vi "CTRE_Phoenix_CANCoder_GetVelocity.vi"(8 "error in":errorcluster, 11 "CTRE_CANcoder_DeviceRef":T1) -> (0 "error out":errorcluster, 2 "Velocity":dbl format="%.2f", 3 "CTRE_CANcoder_DeviceRef":T1)   [LabVIEW 2019]
doc: "Returns the velocity of the CANcoder."
uses:
  <vilib>/Rock Robotics/WPI/ThirdParty/Phoenix-LabVIEW/CANCoder/Controls/CTRE_Phoenix_CANcoder_DeviceRef.ctl
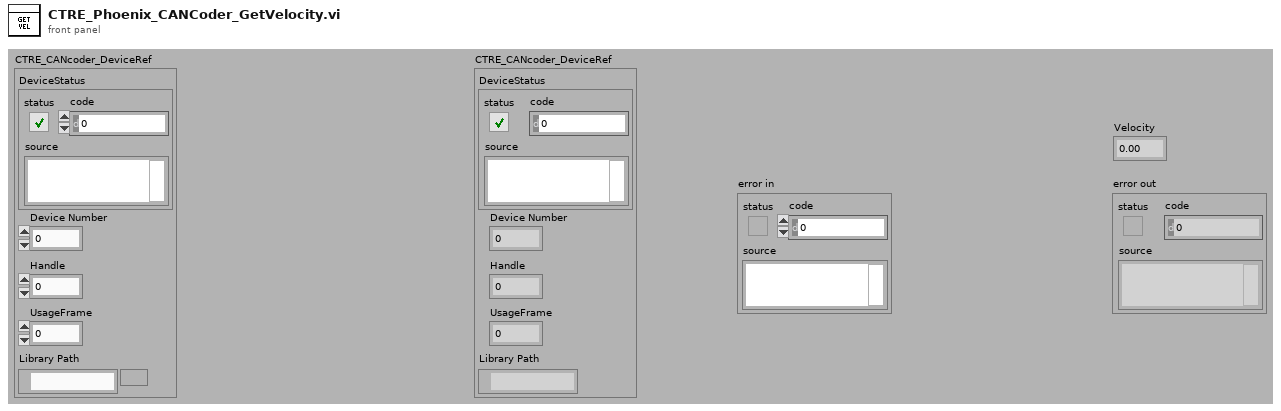
[diagram p1: front panel]
types:
  T1 = typedef "CTRE_Phoenix_CANcoder_DeviceRef.ctl" = cluster{"DeviceStatus":errorcluster, "Device Number":u8, "Handle":u64, "UsageFrame":u32, "Library Path":path}
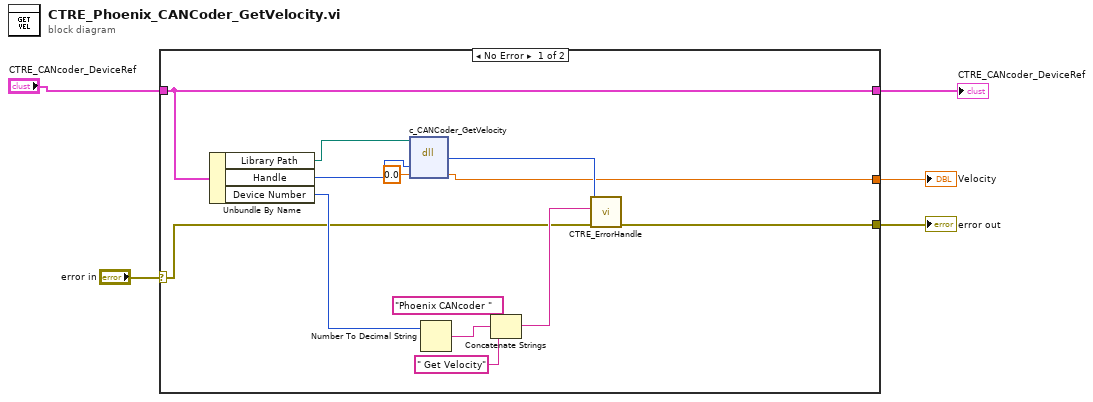
[diagram p0: block diagram]
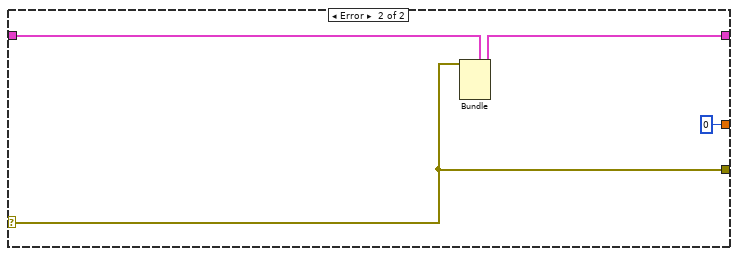
[diagram p2: hidden frame]
diagram:
  n1 = case shown="No Error" "error in" {
    selector: "error in" -> [w6 w21]
    tunnel: "CTRE_CANcoder_DeviceRef" -> [w10 w22]
    tunnel: [w17 w21] -> w5
    tunnel: [w10 w20] -> w1
    tunnel: [w11 0 ("percentOutput")] -> w3
    frame No Error {
      n2 = Unbundle By Name(w10) -> ("Library Path"=w8:path, "Handle"=w7:u64, "Device Number"=w9:u8)
      n3 = dll-call lib="?" fn="c_CANCoder_GetVelocity"(path in=w8, "handle"=w7, "velocity"=0.0 ("appliedThrottle")) -> ("return type"=w13:i32, "velocity"=w11:dbl)  [unwired: 3 in, 2 out]
      n4 = Number To Decimal String(number=w9) -> (decimal integer string=w15:string)  [unwired: 1 in]
      n5 = Concatenate Strings("Phoenix CANcoder " ("string"), w15, " Get Velocity" ("string")) -> (w12:string)
      n6 = call <vilib>:"CTRE_ErrorHandle.vi"("error in"=w6, "origin"=w12, "code"=w13) -> ("error out"=w17:errorcluster)  [unwired: 8 in]
    }
    frame Error {
      n7 = Bundle(cluster=w22, "DeviceStatus"=w21) -> (w20:T1)  [unwired: 4 in]
    }
  }
  "Velocity" <- w3
  "error out" <- w5
  "CTRE_CANcoder_DeviceRef" <- w1
